vi "load_sat_data.vi"() -> (0 "sat(U_nom)":dbl[](array[numeric]), 1 "U_nom":dbl[](array[numeric]), 2 "wsp":dbl[](array[numeric]), 3 "dps":dbl[](array[numeric]), 4 "N_hyst":i32)   [LabVIEW 2017, in "Sat_Hyst_TestCase.lvclass"]
uses:
  Sat_Hyst_TestCase.lvclass
  <vilib>/Utility/file.llb/Read Delimited Spreadsheet (DBL).vi
panel:
  out "all rows":dbl[][](array[numeric])
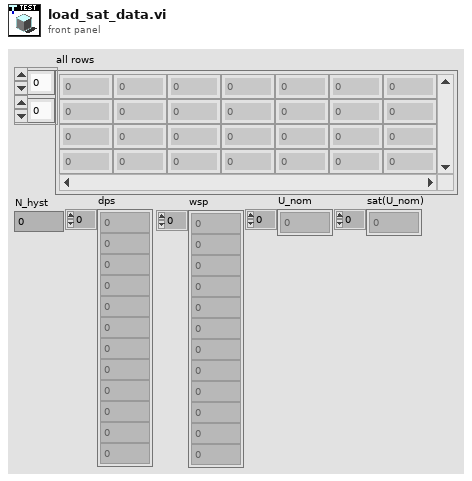
[diagram p1: front panel]
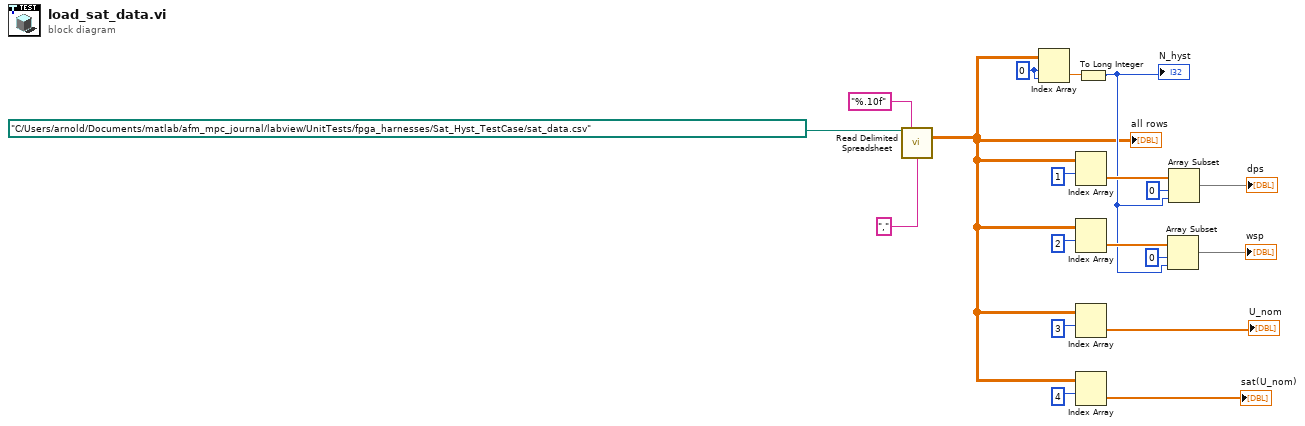
[diagram p0: block diagram]
diagram:
  w16 = 0 ("index (row)")
  n1 = call-poly <vilib>:"Read Delimited Spreadsheet.vi"("file path (dialog if empty)"=path "C:/Users/arnold/Documents/matlab/afm_mpc_journal/labview/UnitTests/fpga_harnesses/Sat_Hyst_TestCase/sat_data.csv" ("Path"), "format (%.3f)"="%.10f", "delimiter (\\t)"="," ("delimiter (\\t)")) -> ("all rows"=w3:dbl[][])  [unwired: 7 in, 5 out]
  "all rows" <- w3
  n2 = Index Array(array=w3, index (row)=w16, index (col)=w16) -> (element=w9:dbl)
  n3 = Index Array(array=w3, index (row)=1) -> (element=w14:dbl[])  [unwired: 1 in]
  n4 = Index Array(array=w3, index (row)=2) -> (element=w11:dbl[])  [unwired: 1 in]
  n5 = Index Array(array=w3, index (row)=3) -> (element=→"U_nom":dbl[])  [unwired: 1 in]
  n6 = Index Array(array=w3, index (row)=4) -> (element=→"sat(U_nom)":dbl[])  [unwired: 1 in]
  n7 = To Long Integer(number=w9) -> (32bit integer=w8:i32)
  "N_hyst" <- w8
  n8 = Array Subset(array=w11, index=0, length=w8) -> (→"wsp":dbl[])
  n9 = Array Subset(array=w14, index=0, length=w8) -> (→"dps":dbl[])
